vi "Teleop.vi"(10 "Match Info":T1={"Autonomous Elapsed Seconds"=0.0, "TeleOp Elapsed Seconds"=0.0, "Disabled Elapsed Seconds"=0.0, "Visited Autonomous"=FALSE, "Visited TeleOp"=FALSE, "Visited Disabled"=FALSE, "Autonomous Settings"={"Autonomous Style"=enum."Independent", "VI Refnum"=refnum}}, 11 "Call Context":T2) -> ()   [LabVIEW 2014]
doc: "This VI is called for each TeleOp packet received from the DS where the robot is not disabled. It is often used to read from the joysticks and update I/O or to update setpoints for timed control loops. It should complete and return within 20 milliseconds or it may miss DS packets."
uses:
  <vilib>/Rock Robotics/WPI/DriverStation/WPI_DriverStationDerivedRobotMode.ctl
  <vilib>/Rock Robotics/WPI/DriverStation/WPI_DriverStationMatch Info.ctl
  <vilib>/Rock Robotics/Network Tables/SD Read Boolean.vi
  <vilib>/Rock Robotics/Network Tables/SD Read Number.vi
  Global Var.vi
  <vilib>/Rock Robotics/WPI/Joystick/WPI_JoystickGetSetRefNum.vi
  <vilib>/addons/control/pid/pid.llb/PID (DBL).vi
  <vilib>/Rock Robotics/WPI/RobotDrive/WPI_RobotDriveGetSetRefNum.vi
  Global 1.vi
  <vilib>/Rock Robotics/Network Tables/SD Write Number.vi
  <vilib>/Rock Robotics/Network Tables/SD Write Boolean Array.vi
  <vilib>/Rock Robotics/Network Tables/SD Write Numeric Array.vi
  <vilib>/Rock Robotics/WPI/RobotDrive/WPI_RobotDriveMecanumDrive_Cartesian.vi
  <vilib>/addons/control/pid/NI_PID_pid.lvlib
panel:
  out "Sample Slider 0":dbl(slide) scale=0.0..5.0
  out "Sample Boolean 1":bool
  out "Sample Boolean 0":bool
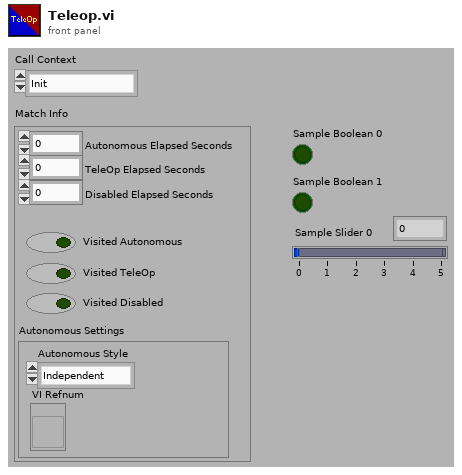
[diagram p1: front panel]
types:
  T1 = typedef "WPI_DriverStationMatch Info.ctl" = cluster{"Autonomous Elapsed Seconds":dbl, "TeleOp Elapsed Seconds":dbl, "Disabled Elapsed Seconds":dbl, "Visited Autonomous":bool, "Visited TeleOp":bool, "Visited Disabled":bool, "Autonomous Settings":cluster{"Autonomous Style":enum16{"Iterative", "Independent"}, "VI Refnum":refnum<vi>}}
  T2 = typedef "WPI_DriverStationDerivedRobotMode.ctl" = enum16{"Init", "Execute", "Stop"}
  T3 = typedef "WPI_JoystickDevRef.ctl" = cluster{"Device":T4}
  T4 = typedef "WPI_JoystickDeviceEnum.ctl" = enum16{"USB 0", "USB 1", "USB 2", "USB 3", "USB 4", "USB 5"}
  T5 = cluster{"Buttons[0]":bool, "Buttons[1]":bool, "Buttons[2]":bool, "Buttons[3]":bool, "Buttons[4]":bool, "Buttons[5]":bool, "Buttons[6]":bool, "Buttons[7]":bool, "Buttons[8]":bool, "Buttons[9]":bool, "Buttons[10]":bool, "Buttons[11]":bool}
  T6 = typedef "WPI_MotorControlDeviceRef.ctl" = cluster{"DeviceStatus":errorcluster, "Type":T7, "PWM":cluster{"Controller":T8, "PWM Channel":T9, "DeadBand":T10}, "CAN":cluster{"Device Number":u8, "Control Mode":T11, "Semaphore":T12, "Max Vout":dbl, "TalonSRX Control Mode":T13}, "Invert":bool, "TransformRef":T14, "InvTransformRef":T14}
  T7 = typedef "WPI_MotorControlType.ctl" = enum16{"PWM", "CAN", "CANTalonSRX"}
  T8 = typedef "FPGA_TypedefDigitalModule.ctl" = enum16{"Controller 1"}
  T9 = typedef "FPGA_DIOPWMChannel.ctl" = enum8{"PWM 0", "PWM 1", "PWM 2", "PWM 3", "PWM 4", "PWM 5", "PWM 6", "PWM 7", "PWM 8", "PWM 9", "PWM MXP 0", "PWM MXP 1", "PWM MXP 2", "PWM MXP 3", "PWM MXP 4", "PWM MXP 5", "PWM MXP 6", "PWM MXP 7", "PWM MXP 8", "PWM MXP 9", "Invalid"}
  T10 = typedef "WPI_PWMDeadband.ctl" = cluster{"Name":string, "maxPositivePwm":i32, "minPositivePwm":i32, "centerPwm":i32, "maxNegativePwm":i32, "minNegativePwm":i32, "angularRange":u16}
  T11 = typedef "WPI_CANJaguar_ControlMode.ctl" = enum8{"Percent VBus", "Current", "Speed", "Position", "Voltage"}
  T12 = typedef "Semaphore RefNum" = refnum<k1>
  T13 = typedef "WPI_CANTalonSRX_APIControlMode.ctl" = enum8{"Percent VBus", "Speed", "Position", "Slave", "Unchanged / Invalid"}
  T14 = typedef "WPI_PWMTransform_ConPane.ctl" = refnum<vi>
  T15 = typedef "WPI_RobotDriveDevRef.ctl" = cluster{"DevStatus":errorcluster, "Motors[]":T6[], "Square Inputs":bool, "Max Output":dbl}
  T16 = cluster{"proportional gain (Kc)":dbl, "integral time (Ti, min)":dbl, "derivative time (Td, min)":dbl}
  T17 = cluster{"Axes[0]":dbl, "Axes[1]":dbl, "Axes[2]":dbl, "Axes[3]":dbl, "Axes[4]":dbl, "Axes[5]":dbl, "Axes[6]":dbl, "Axes[7]":dbl, "Axes[8]":dbl, "Axes[9]":dbl, "Axes[10]":dbl, "Axes[11]":dbl}
  T18 = typedef "WPI_DigitalInputDevRef.ctl" = cluster{"DevStatus":errorcluster, "DIO Channel":T19, "Controller":T8}
  T19 = typedef "FPGA_DIOChannel.ctl" = enum8{"DIO 0", "DIO 1", "DIO 2", "DIO 3", "DIO 4", "DIO 5", "DIO 6", "DIO 7", "DIO 8", "DIO 9", "DIO MXP 0", "DIO MXP 1", "DIO MXP 2", "DIO MXP 3", "DIO MXP 4", "DIO MXP 5", "DIO MXP 6", "DIO MXP 7", "DIO MXP 8", "DIO MXP 9", "DIO MXP 10", "DIO MXP 11", "DIO MXP 12", "DIO MXP 13", "DIO MXP 14", "DIO MXP 15", "Invalid"}
  T20 = typedef "WPI_EncoderDevRef.ctl" = cluster{"DevStatus":errorcluster, "EncoderIndex":T21, "CounterIndex":T22, "DistancePerCount":dbl, "Decoding Type":T23}
  T21 = typedef "FPGA_EncoderIdx.ctl" = enum8{"Enc 0", "Enc 1", "Enc 2", "Enc 3", "Enc 4", "Enc 5", "Enc 6", "Enc 7", "Invalid"}
  T22 = typedef "FPGA_CounterCtrSystemIndex.ctl" = enum8{"Ctr 0", "Ctr 1", "Ctr 2", "Ctr 3", "Ctr 4", "Ctr 5", "Ctr 6", "Ctr 7", "Invalid"}
  T23 = typedef "WPI_EncoderType.ctl" = enum16{"1x", "2x", "4x"}
  T24 = cluster{"Buttons[0]":bool, "Buttons[1]":bool, "Buttons[2]":bool, "Buttons[3]":bool, "Buttons[4]":bool, "Buttons[5]":bool, "Buttons[6]":bool, "Buttons[7]":bool, "Buttons[8]":bool}
  T25 = typedef "WPI_GyroDevRef.ctl" = cluster{"DevStatus":errorcluster, "Analog Module":T26, "Analog Channel":T27, "Offset":dbl, "Gain (VoltsPerDegree/Second)":dbl}
  T26 = typedef "FPGA_TypedefAnalogModule.ctl" = enum16{"Controller 1"}
  T27 = typedef "FPGA_AIChannel.ctl" = enum8{"AI 0", "AI 1", "AI 2", "AI 3", "AI MXP 0", "AI MXP 1", "AI MXP 2", "AI MXP 3", "Invalid"}
  T28 = cluster{"Axes[0]":dbl, "Axes[1]":dbl, "Axes[2]":dbl, "Axes[3]":dbl, "Axes[4]":dbl, "Axes[5]":dbl, "Axes[6]":dbl, "Axes[7]":dbl, "Axes[8]":dbl}
  T29 = typedef "WPI_ServoDeviceRef.ctl" = cluster{"DeviceStatus":errorcluster, "Controller":T8, "PWM Channel":T9, "DeadBand":T10}
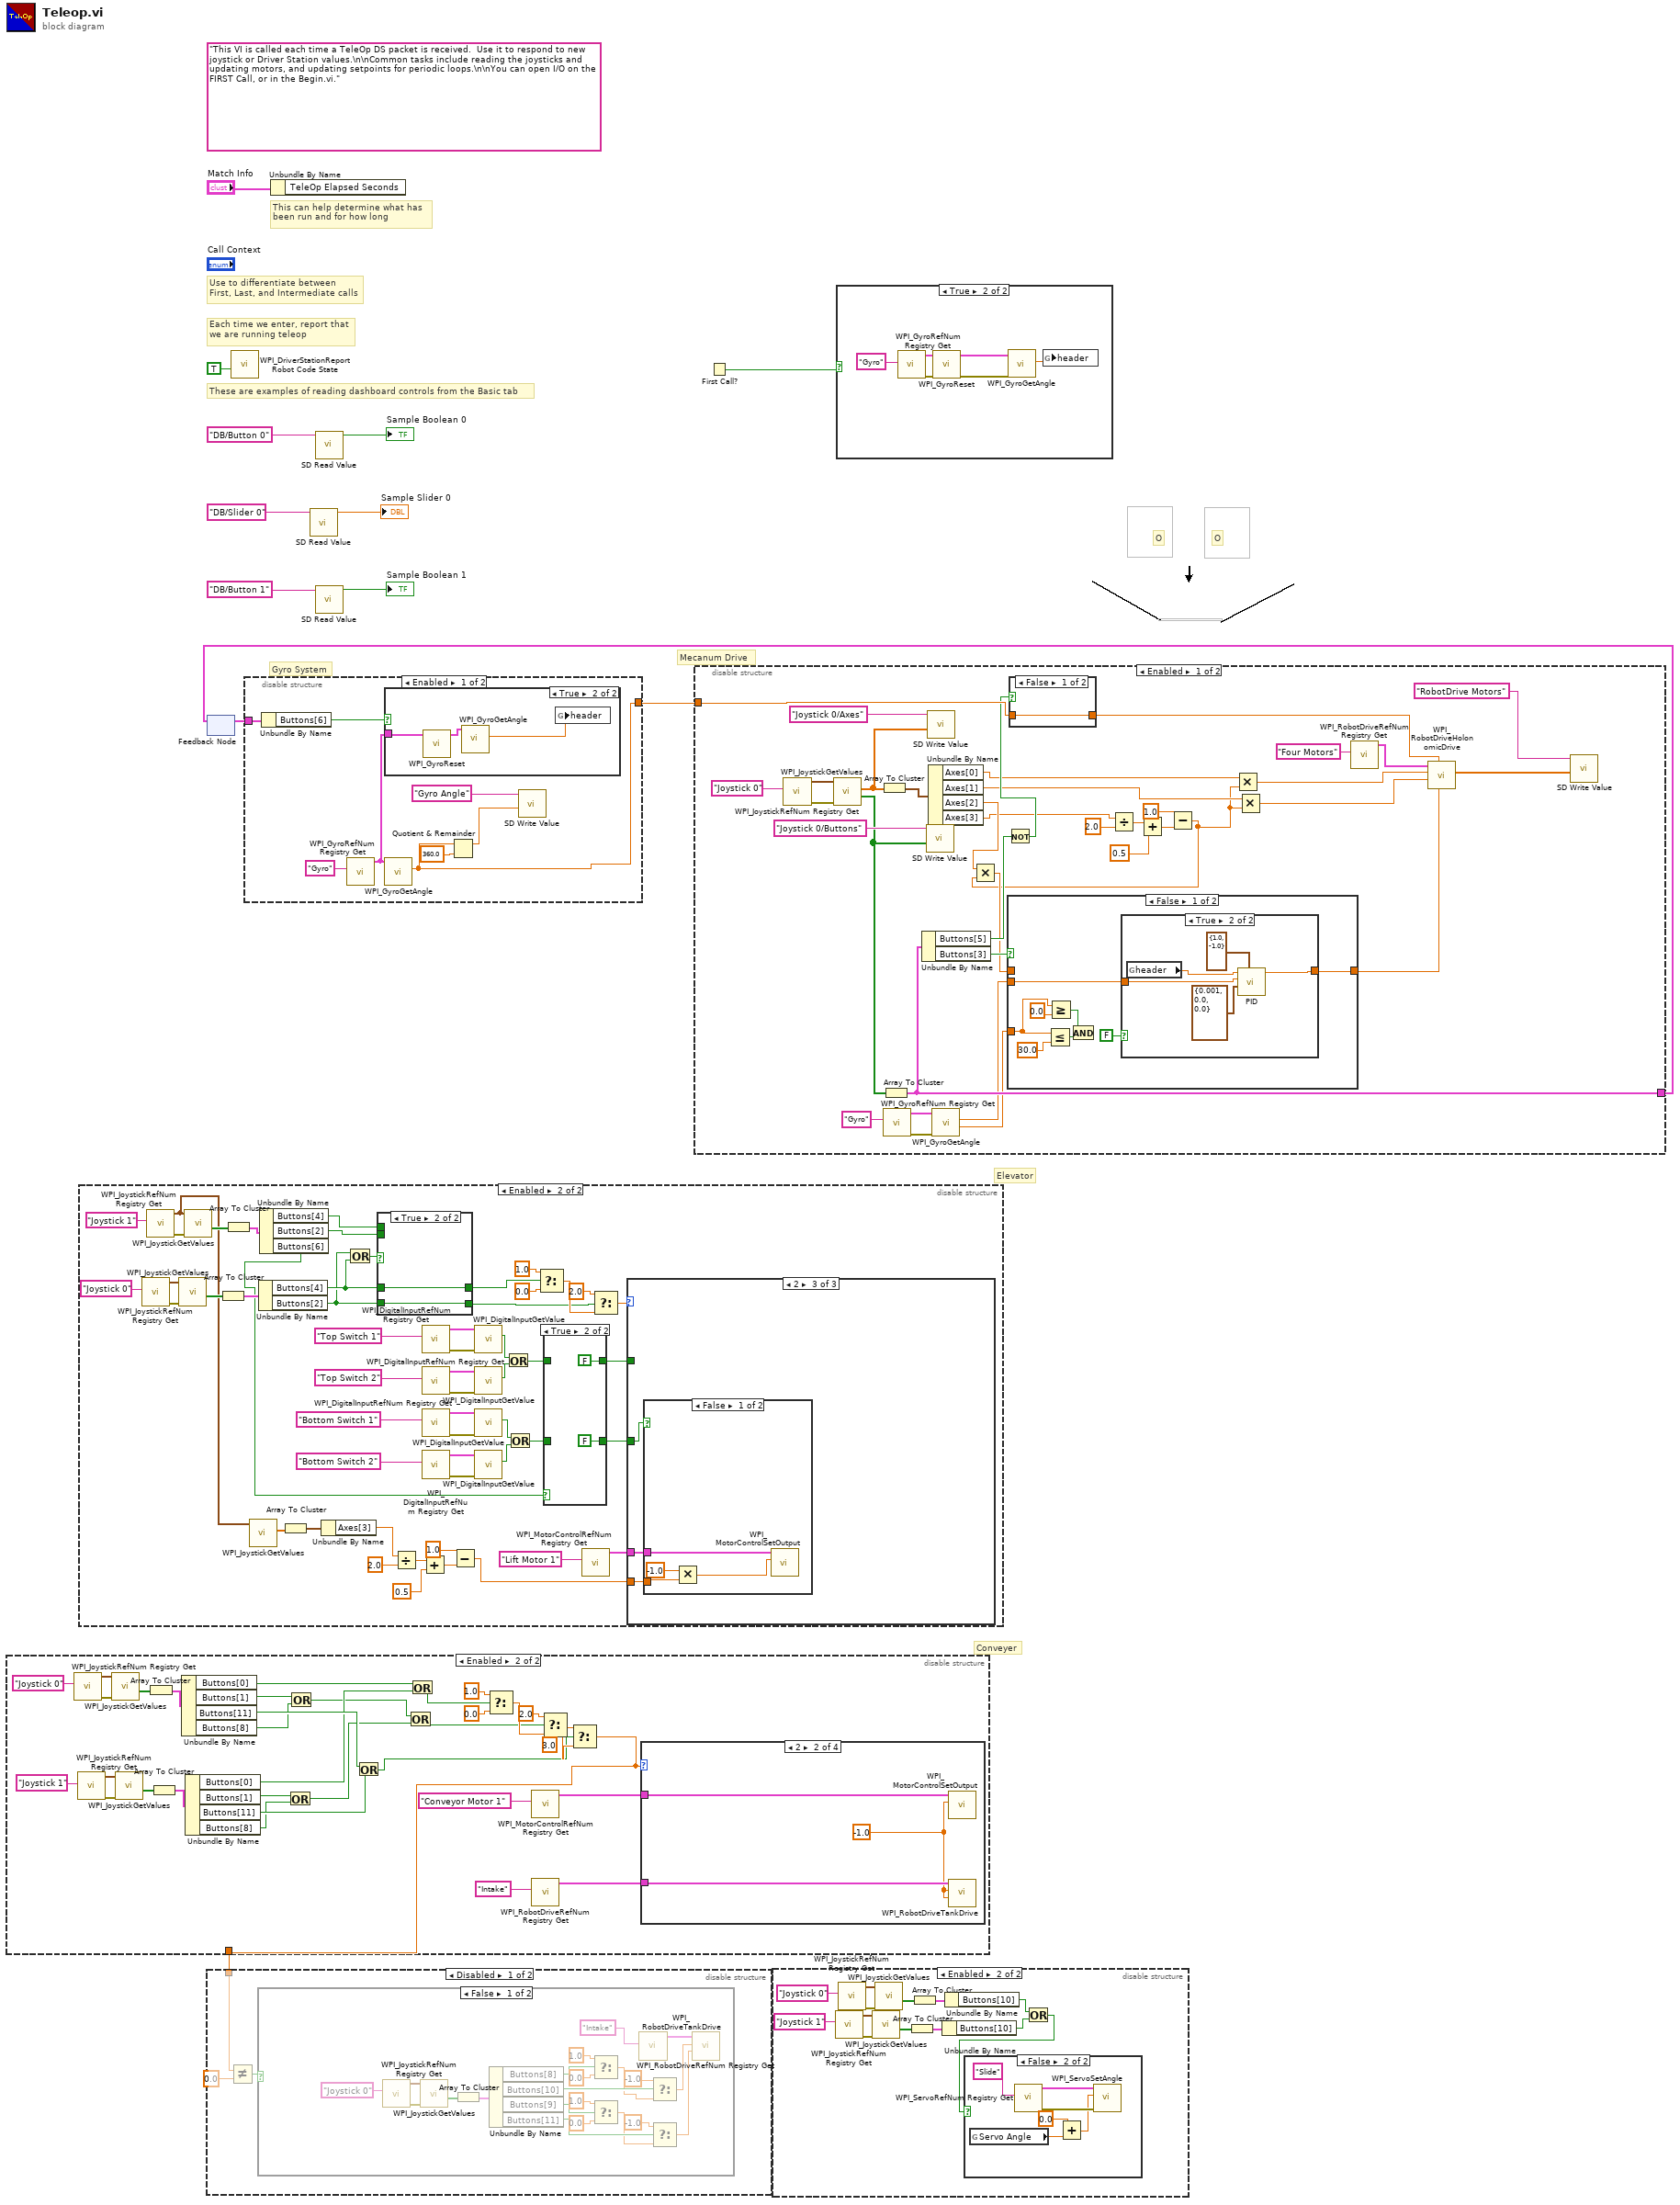
[diagram p0: block diagram]
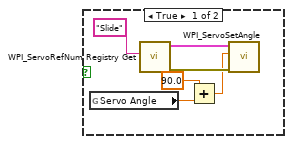
[diagram p3: hidden frame]
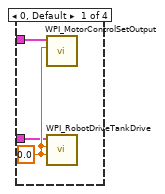
[diagram p8: hidden frame]
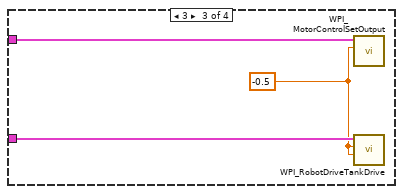
[diagram p9: hidden frame]
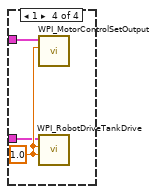
[diagram p10: hidden frame]
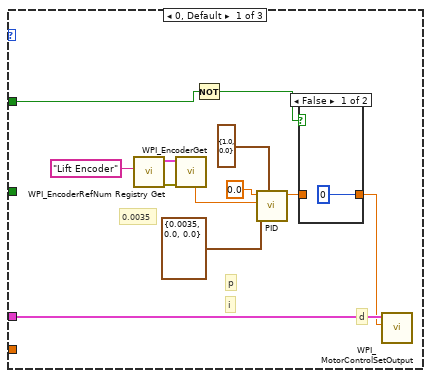
[diagram p14: hidden frame]
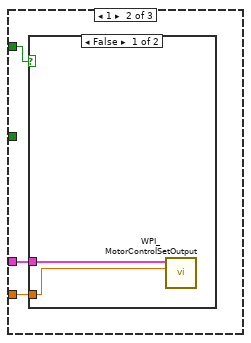
[diagram p16: hidden frame]
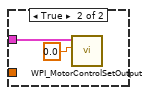
[diagram p17: hidden frame]
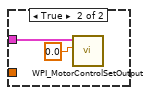
[diagram p18: hidden frame]
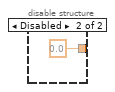
[diagram p20: hidden frame]
diagram:
  (unwired) "This VI is called each time a TeleOp DS packet is received.  Use it to respond to new joystick or Driver Station values.\n\nCommon tasks include reading the joysticks and updating motors, and updating setpoints for periodic loops.\n\nYou can open I/O on the FIRST Call, or in the Begin.vi."
  # "O"
  # "O"
  # "Conveyer"
  # "Gyro System"
  # "Mecanum Drive"
  # "Elevator"
  # "These are examples of reading dashboard controls from the Basic tab"
  # "Each time we enter, report that\nwe are running teleop"
  # "Use to differentiate between\nFirst, Last, and Intermediate calls"
  # "This can help determine what has\nbeen run and for how long"
  n1 = disable-structure shown="Enabled" {
    disable-tunnel: [_ w34] -> w1
    frame Disabled {
    }
    frame Enabled {
      n2 = call <vilib>:"WPI_JoystickRefNum Registry Get.vi"("refnum name"="Joystick 0") -> ("error out"=w43:errorcluster, "JoystickDevRef"=w44:T3)  [unwired: 9 in]
      n3 = call <vilib>:"WPI_JoystickRefNum Registry Get.vi"("refnum name"="Joystick 1") -> ("error out"=w29:errorcluster, "JoystickDevRef"=w30:T3)  [unwired: 9 in]
      n4 = call <vilib>:"WPI_JoystickGetValues.vi"("error in (no error)"=w43, "JoystickDevRef"=w44) -> ("Buttons"=w40:bool[])  [unwired: 5 in, 4 out]
      n5 = call <vilib>:"WPI_JoystickGetValues.vi"("error in (no error)"=w29, "JoystickDevRef"=w30) -> ("Buttons"=w28:bool[])  [unwired: 5 in, 4 out]
      n6 = Array To Cluster(array=w40) -> (cluster=w39:T5)
      n7 = Array To Cluster(array=w28) -> (cluster=w27:T5)
      n8 = Unbundle By Name(w39) -> ("Buttons[0]"=w20:bool, "Buttons[1]"=w17:bool, "Buttons[11]"=w24:bool, "Buttons[8]"=w18:bool)
      n9 = Unbundle By Name(w27) -> ("Buttons[0]"=w21:bool, "Buttons[1]"=w16:bool, "Buttons[11]"=w26:bool, "Buttons[8]"=w15:bool)
      n10 = Or(x=w16, y=w15) -> (x .or. y?=w14:bool)
      n11 = Or(x=w17, y=w18) -> (x .or. y?=w19:bool)
      n12 = Or(x=w24, y=w26) -> (x .or. y?=w25:bool)
      n13 = Or(x=w19, y=w14) -> (x .or. y?=w23:bool)
      n14 = Or(x=w20, y=w21) -> (x .or. y?=w22:bool)
      n15 = Select(t=1.0, s=w22, f=0.0) -> (s? t:f=w35:dbl)
      n16 = call <vilib>:"WPI_MotorControlRefNum Registry Get.vi"("refnum name"="Conveyor Motor 1") -> ("MotorControlDevRef"=w41:T6)  [unwired: 9 in, 1 out]
      n17 = call <vilib>:"WPI_RobotDriveRefNum Registry Get.vi"("refnum name"="Intake") -> ("RobotDriveDevRef"=w42:T15)  [unwired: 9 in, 1 out]
      n18 = Select(t=2.0, s=w23, f=w35) -> (s? t:f=w33:dbl)
      n19 = Select(t=3.0 ("f"), s=w25, f=w33) -> (s? t:f=w34:dbl)
      n20 = case shown="2" w34 {
        tunnel: w42 -> [w48 w52 w55 w57]
        tunnel: w41 -> [w50 w53 w56 w59]
        frame 0, Default {
          w49 = 0.0 ("Output")
          n21 = call <vilib>:"WPI_MotorControlSetOutput.vi"("Output"=w49, "MotorControlDevRef"=w50) -> ()  [unwired: 7 in, 3 out]
          n22 = call <vilib>:"WPI_RobotDriveTankDrive.vi"("Right axis value"=w49, "Left axis value"=w49, "RobotDriveDevRef"=w48) -> ()  [unwired: 6 in, 3 out]
        }
        frame 2 {
          w51 = -1.0
          n23 = call <vilib>:"WPI_MotorControlSetOutput.vi"("Output"=w51, "MotorControlDevRef"=w53) -> ()  [unwired: 7 in, 3 out]
          n24 = call <vilib>:"WPI_RobotDriveTankDrive.vi"("Right axis value"=w51, "Left axis value"=w51, "RobotDriveDevRef"=w52) -> ()  [unwired: 6 in, 3 out]
        }
        frame 3 {
          w54 = -0.5
          n25 = call <vilib>:"WPI_MotorControlSetOutput.vi"("Output"=w54, "MotorControlDevRef"=w56) -> ()  [unwired: 7 in, 3 out]
          n26 = call <vilib>:"WPI_RobotDriveTankDrive.vi"("Right axis value"=w54, "Left axis value"=w54, "RobotDriveDevRef"=w55) -> ()  [unwired: 6 in, 3 out]
        }
        frame 1 {
          w58 = 1.0 ("Output")
          n27 = call <vilib>:"WPI_MotorControlSetOutput.vi"("Output"=w58, "MotorControlDevRef"=w59) -> ()  [unwired: 7 in, 3 out]
          n28 = call <vilib>:"WPI_RobotDriveTankDrive.vi"("Right axis value"=w58, "Left axis value"=w58, "RobotDriveDevRef"=w57) -> ()  [unwired: 6 in, 3 out]
        }
      }
    }
  }
  n29 = disable-structure shown="Enabled" {
    frame Disabled {
    }
    frame Enabled {
      n30 = call <vilib>:"WPI_JoystickRefNum Registry Get.vi"("refnum name"="Joystick 0") -> ("error out"=w110:errorcluster, "JoystickDevRef"=w111:T3)  [unwired: 9 in]
      n31 = call <vilib>:"WPI_JoystickRefNum Registry Get.vi"("refnum name"="Joystick 1") -> ("error out"=w84:errorcluster, "JoystickDevRef"=w74:T3)  [unwired: 9 in]
      n32 = call <vilib>:"WPI_JoystickGetValues.vi"("error in (no error)"=w110, "JoystickDevRef"=w111) -> ("Buttons"=w102:bool[])  [unwired: 5 in, 4 out]
      n33 = call <vilib>:"WPI_JoystickGetValues.vi"("error in (no error)"=w84, "JoystickDevRef"=w74) -> ("Buttons"=w83:bool[])  [unwired: 5 in, 4 out]
      n34 = Array To Cluster(array=w102) -> (cluster=w101:T5)
      n35 = Array To Cluster(array=w83) -> (cluster=w82:T5)
      n36 = call <vilib>:"WPI_JoystickGetValues.vi"("JoystickDevRef"=w74) -> ("Axes"=w72:dbl[])  [unwired: 6 in, 4 out]
      n37 = Unbundle By Name(w101) -> ("Buttons[4]"=w76:bool, "Buttons[2]"=w75:bool)
      n38 = Unbundle By Name(w82) -> ("Buttons[4]"=w79:bool, "Buttons[2]"=w78:bool, "Buttons[6]"=w60:bool)
      n39 = Array To Cluster(array=w72) -> (cluster=w73:T17)
      n40 = Unbundle By Name(w73) -> ("Axes[3]"=w67:dbl)
      n41 = Or(x=w75, y=w76) -> (x .or. y?=w77:bool)
      n42 = case shown="True" w77 {
        tunnel: w76 -> [_ w121]
        tunnel: [w119 w121] -> w81
        tunnel: w75 -> [_ w120]
        tunnel: [w118 w120] -> w80
        tunnel: w79 -> [w119 _]
        tunnel: w78 -> [w118 _]
        frame False {
        }
        frame True {
        }
      }
      n43 = Divide(x=w67, y=2.0) -> (x/y=w70:dbl)
      n44 = Add(x=w70, y=0.5) -> (x+y=w69:dbl)
      n45 = call <vilib>:"WPI_DigitalInputRefNum Registry Get.vi"("refnum name"="Top Switch 1") -> ("error out"=w107:errorcluster, "DigitalInputDevRef"=w106:T18)  [unwired: 9 in]
      n46 = call <vilib>:"WPI_DigitalInputRefNum Registry Get.vi"("refnum name"="Top Switch 2") -> ("error out"=w91:errorcluster, "DigitalInputDevRef"=w90:T18)  [unwired: 9 in]
      n47 = call <vilib>:"WPI_DigitalInputRefNum Registry Get.vi"("refnum name"="Bottom Switch 1") -> ("error out"=w94:errorcluster, "DigitalInputDevRef"=w93:T18)  [unwired: 9 in]
      n48 = call <vilib>:"WPI_DigitalInputRefNum Registry Get.vi"("refnum name"="Bottom Switch 2") -> ("error out"=w104:errorcluster, "DigitalInputDevRef"=w103:T18)  [unwired: 9 in]
      n49 = Subtract(x=1.0, y=w69) -> (x-y=w65:dbl)
      n50 = call <vilib>:"WPI_DigitalInputGetValue.vi"("error in (no error)"=w107, "DigitalInputDevRef"=w106) -> ("Value"=w89:bool)  [unwired: 7 in, 2 out]
      n51 = call <vilib>:"WPI_DigitalInputGetValue.vi"("error in (no error)"=w91, "DigitalInputDevRef"=w90) -> ("Value"=w88:bool)  [unwired: 7 in, 2 out]
      n52 = call <vilib>:"WPI_DigitalInputGetValue.vi"("error in (no error)"=w94, "DigitalInputDevRef"=w93) -> ("Value"=w86:bool)  [unwired: 7 in, 2 out]
      n53 = call <vilib>:"WPI_DigitalInputGetValue.vi"("error in (no error)"=w104, "DigitalInputDevRef"=w103) -> ("Value"=w87:bool)  [unwired: 7 in, 2 out]
      n54 = Or(x=w89, y=w88) -> (x .or. y?=w61:bool)
      n55 = Or(x=w86, y=w87) -> (x .or. y?=w63:bool)
      n56 = Select(t=1.0, s=w81, f=0.0) -> (s? t:f=w96:dbl)
      n57 = case shown="True" w60 {
        tunnel: [w115 FALSE] -> w64
        tunnel: w63 -> [w115 _]
        tunnel: [w114 FALSE] -> w62
        tunnel: w61 -> [w114 _]
        frame False {
        }
        frame True {
        }
      }
      n58 = call <vilib>:"WPI_MotorControlRefNum Registry Get.vi"("refnum name"="Lift Motor 1") -> ("MotorControlDevRef"=w109:T6)  [unwired: 9 in, 1 out]
      n59 = Select(t=2.0, s=w80, f=w96) -> (s? t:f=w97:dbl)
      n60 = case shown="2" w97 {
        tunnel: w109 -> [w127 w138 w145]
        tunnel: w62 -> [w123 w137 _]
        tunnel: w64 -> [_ _ w144]
        tunnel: w65 -> [_ w136 w143]
        frame 0, Default {
          # "0.0035"
          # "d"
          # "i"
          # "p"
          n61 = call <vilib>:"WPI_EncoderRefNum Registry Get.vi"("refnum name"="Lift Encoder") -> ("error out"=w132:errorcluster, "EncoderDevRef"=w133:T20)  [unwired: 9 in]
          n62 = call <vilib>:"WPI_EncoderGet.vi"("error in (no error)"=w132, "EncoderDevRef"=w133) -> ("Rate"=w129:dbl)  [unwired: 4 in, 5 out]
          n63 = Not(x=w123) -> (.not. x?=w124:bool)
          n64 = call-poly <vilib>:"PID.vi"("output range"=cluster{"output high":dbl, "output low":dbl} {"output high"=1.0, "output low"=0.0}, "PID gains"=T16 {"proportional gain (Kc)"=0.0035, "integral time (Ti, min)"=0.0, "derivative time (Td, min)"=0.0}, "process variable"=w129, "setpoint"=0.0 ("Output")) -> ("output"=w125:dbl)  [unwired: 6 in, 1 out]
          n65 = case shown="False" w124 {
            tunnel: [0 w135] -> w126
            tunnel: w125 -> [_ w135]
            frame False {
            }
            frame True {
            }
          }
          n66 = call <vilib>:"WPI_MotorControlSetOutput.vi"("Output"=w126, "MotorControlDevRef"=w127) -> ()  [unwired: 7 in, 3 out]
        }
        frame 1 {
          n67 = case shown="False" w137 {
            tunnel: w138 -> [w140 w141]
            tunnel: w136 -> [w139 _]
            frame False {
              n68 = call <vilib>:"WPI_MotorControlSetOutput.vi"("Output"=w139, "MotorControlDevRef"=w140) -> ()  [unwired: 7 in, 3 out]
            }
            frame True {
              n69 = call <vilib>:"WPI_MotorControlSetOutput.vi"("Output"=0.0, "MotorControlDevRef"=w141) -> ()  [unwired: 7 in, 3 out]
            }
          }
        }
        frame 2 {
          n70 = case shown="False" w144 {
            tunnel: w145 -> [w149 w150]
            tunnel: w143 -> [w148 _]
            frame False {
              n71 = Multiply(x=-1.0, y=w148) -> (x*y=w147:dbl)
              n72 = call <vilib>:"WPI_MotorControlSetOutput.vi"("Output"=w147, "MotorControlDevRef"=w149) -> ()  [unwired: 7 in, 3 out]
            }
            frame True {
              n73 = call <vilib>:"WPI_MotorControlSetOutput.vi"("Output"=0.0, "MotorControlDevRef"=w150) -> ()  [unwired: 7 in, 3 out]
            }
          }
        }
      }
    }
  }
  n74 = feedback #1() -> (w5:T24)  [unwired: 1 in]
  n75 = disable-structure shown="Disabled" {
    disable-tunnel: w1 -> [w152 _]
    frame Disabled {
      n76 = Not Equal?(x=w152, y=0.0) -> (x != y?=w154:bool)
      n77 = case shown="False" w154 {
        frame False {
          n78 = call <vilib>:"WPI_JoystickRefNum Registry Get.vi"("refnum name"="Joystick 0") -> ("error out"=w172:errorcluster, "JoystickDevRef"=w171:T3)  [unwired: 9 in]
          n79 = call <vilib>:"WPI_JoystickGetValues.vi"("error in (no error)"=w172, "JoystickDevRef"=w171) -> ("Buttons"=w170:bool[])  [unwired: 5 in, 4 out]
          n80 = Array To Cluster(array=w170) -> (cluster=w169:T5)
          n81 = Unbundle By Name(w169) -> ("Buttons[8]"=w168:bool, "Buttons[10]"=w165:bool, "Buttons[9]"=w161:bool, "Buttons[11]"=w162:bool)
          n82 = Select(t=1.0, s=w168, f=0.0) -> (s? t:f=w157:dbl)
          n83 = Select(t=1.0, s=w161, f=0.0) -> (s? t:f=w158:dbl)
          n84 = call <vilib>:"WPI_RobotDriveRefNum Registry Get.vi"("refnum name"="Intake") -> ("RobotDriveDevRef"=w174:T15)  [unwired: 9 in, 1 out]
          n85 = Select(t=-1.0 ("f"), s=w165, f=w157) -> (s? t:f=w159:dbl)
          n86 = Select(t=-1.0 ("f"), s=w162, f=w158) -> (s? t:f=w160:dbl)
          n87 = call <vilib>:"WPI_RobotDriveTankDrive.vi"("Right axis value"=w160, "Left axis value"=w159, "RobotDriveDevRef"=w174) -> ()  [unwired: 6 in, 3 out]
        }
        frame True {
        }
      }
    }
    frame Enabled {
    }
  }
  n88 = call <vilib>:"WPI_DriverStationReport Robot Code State.vi"("TeleOp"=TRUE ("Autonomous")) -> ()  [unwired: 10 in, 1 out]
  n89 = disable-structure shown="Enabled" {
    disable-tunnel: w5 -> [w180 _]
    disable-tunnel: [w176 0.0] -> w4
    frame Enabled {
      n90 = Unbundle By Name(w180) -> ("Buttons[6]"=w179:bool)
      n91 = call <vilib>:"WPI_GyroRefNum Registry Get.vi"("refnum name"="Gyro") -> ("GyroDevRef"=w178:T25)  [unwired: 9 in, 1 out]
      n92 = case shown="True" w179 {
        tunnel: w178 -> [_ w186]
        frame False {
        }
        frame True {
          n93 = call <vilib>:"WPI_GyroReset.vi"("GyroDevRef"=w186) -> ("GyroDevRef"=w184:T25)  [unwired: 9 in, 1 out]
          n94 = call <vilib>:"WPI_GyroGetAngle.vi"("GyroDevRef"=w184) -> ("Angle"=w185:dbl)  [unwired: 7 in, 3 out]
          n95 = global write "Global Var.vi" "header"(w185) -> ()
        }
      }
      n96 = call <vilib>:"WPI_GyroGetAngle.vi"("GyroDevRef"=w178) -> ("Angle"=w176:dbl)  [unwired: 7 in, 3 out]
      n97 = Quotient & Remainder(x=w176, y=360.0) -> (x-y*floor(x/y)=w177:dbl)  [unwired: 1 out]
      n98 = call-poly <vilib>:"SD Write Value.vi"("Numeric"=w177, "Name"="Gyro Angle") -> ()  [unwired: 8 in, 2 out]
    }
    frame Disabled {
    }
  }
  n99 = Unbundle By Name("Match Info") -> ()  [unwired: 1 out]
  n100 = call-poly <vilib>:"SD Read Value.vi"("Name"="DB/Slider 0" ("refnum name")) -> ("Numeric"=→"Sample Slider 0":dbl)  [unwired: 8 in, 2 out]
  n101 = call-poly <vilib>:"SD Read Value.vi"("Name"="DB/Button 0" ("refnum name")) -> ("Boolean"=→"Sample Boolean 0":bool)  [unwired: 8 in, 2 out]
  n102 = call-poly <vilib>:"SD Read Value.vi"("Name"="DB/Button 1" ("refnum name")) -> ("Boolean"=→"Sample Boolean 1":bool)  [unwired: 8 in, 2 out]
  n103 = disable-structure shown="Enabled" {
    disable-tunnel: [w212 _] -> w3
    disable-tunnel: w4 -> [w205 _]
    frame Enabled {
      n104 = call <vilib>:"WPI_JoystickRefNum Registry Get.vi"("refnum name"="Joystick 0") -> ("error out"=w215:errorcluster, "JoystickDevRef"=w221:T3)  [unwired: 1 in, 8 out]
      n105 = call <vilib>:"WPI_JoystickGetValues.vi"("error in (no error)"=w215, "JoystickDevRef"=w221) -> ("Buttons"=w216:bool[], "Axes"=w214:dbl[])  [unwired: 5 in, 3 out]
      n106 = Array To Cluster(array=w214) -> (cluster=w213:T28)
      n107 = Array To Cluster(array=w216) -> (cluster=w212:T24)
      n108 = call <vilib>:"WPI_GyroRefNum Registry Get.vi"("refnum name"="Gyro") -> ("error out"=w208:errorcluster, "GyroDevRef"=w209:T25)  [unwired: 9 in]
      n109 = Unbundle By Name(w212) -> ("Buttons[5]"=w203:bool, "Buttons[3]"=w210:bool)
      n110 = call-poly <vilib>:"SD Write Value.vi"("Boolean Array"=w216, "Name"="Joystick 0/Buttons") -> ()  [unwired: 8 in, 2 out]
      n111 = call-poly <vilib>:"SD Write Value.vi"("Numeric Array"=w214, "Name"="Joystick 0/Axes") -> ()  [unwired: 8 in, 2 out]
      n112 = Unbundle By Name(w213) -> ("Axes[0]"=w196:dbl, "Axes[1]"=w198:dbl, "Axes[2]"=w194:dbl, "Axes[3]"=w192:dbl)
      n113 = call <vilib>:"WPI_GyroGetAngle.vi"("error in (no error)"=w208, "GyroDevRef"=w209) -> ("Angular Rate"=w206:dbl, "Angle"=w188:dbl)  [unwired: 6 in, 2 out]
      n114 = Not(x=w203) -> (.not. x?=w202:bool)
      n115 = case shown="False" w202 {
        tunnel: w205 -> [w225 _]
        tunnel: [w225 0.0 ("Angle")] -> w204
        frame False {
        }
        frame True {
        }
      }
      n116 = Divide(x=w192, y=2.0) -> (x/y=w200:dbl)
      n117 = Add(x=w200, y=0.5) -> (x+y=w190:dbl)
      n118 = Subtract(x=1.0, y=w190) -> (x-y=w191:dbl)
      n119 = Multiply(x=w194, y=w191) -> (x*y=w193:dbl)
      n120 = case shown="False" w210 {
        tunnel: [w234 w242] -> w211
        tunnel: w193 -> [_ w242]
        tunnel: w188 -> [w233 w241]
        tunnel: w206 -> [w230 _]
        frame False {
          n121 = Less Or Equal?(x=w230, y=30.0) -> (x <= y?=w228:bool)
          n122 = Greater Or Equal?(x=w230, y=0.0 ("x")) -> (x >= y?=w229:bool)
          n123 = And(x=w229, y=w228) -> ()  [unwired: 1 out]
          n124 = case shown="True" FALSE {
            tunnel: [0.0 ("output") w240] -> w234
            tunnel: w233 -> [_ w238]
            frame False {
            }
            frame True {
              n125 = global read "Global Var.vi" "header"() -> (w237:dbl)
              n126 = call-poly <vilib>:"PID.vi"("output range"=cluster{"output high":dbl, "output low":dbl} {"output high"=1.0, "output low"=-1.0}, "PID gains"=T16 {"proportional gain (Kc)"=0.001, "integral time (Ti, min)"=0.0, "derivative time (Td, min)"=0.0}, "process variable"=w238, "setpoint"=w237) -> ("output"=w240:dbl)  [unwired: 6 in, 1 out]
            }
          }
        }
        frame True {
          n127 = global write "Global Var.vi" "header"(w241) -> ()
        }
      }
      n128 = Multiply(x=w196, y=w191) -> (x*y=w195:dbl)
      n129 = Multiply(x=w198, y=w191) -> (x*y=w197:dbl)
      n130 = call <vilib>:"WPI_RobotDriveRefNum Registry Get.vi"("refnum name"="Four Motors") -> ("RobotDriveDevRef"=w223:T15)  [unwired: 1 in, 9 out]
      n131 = call-poly <vilib>:"WPI_RobotDriveHolonomicDrive.vi"("Rotation"=w211, "Gyro Angle"=w204, "Y"=w197, "X"=w195, "RobotDriveDevRef"=w223) -> ("Motor Values"=w217:dbl[])  [unwired: 4 in, 2 out]
      n132 = call-poly <vilib>:"SD Write Value.vi"("Numeric Array"=w217, "Name"="RobotDrive Motors") -> ()  [unwired: 8 in, 2 out]
    }
    frame Disabled {
    }
  }
  n133 = feedback-in #1(w3) -> ()
  n134 = First Call?() -> (First Call?: T/F=w2:bool)
  n135 = disable-structure shown="Enabled" {
    frame Disabled {
    }
    frame Enabled {
      n136 = call <vilib>:"WPI_JoystickRefNum Registry Get.vi"("refnum name"="Joystick 1") -> ("error out"=w253:errorcluster, "JoystickDevRef"=w254:T3)  [unwired: 9 in]
      n137 = call <vilib>:"WPI_JoystickRefNum Registry Get.vi"("refnum name"="Joystick 0") -> ("error out"=w248:errorcluster, "JoystickDevRef"=w249:T3)  [unwired: 9 in]
      n138 = call <vilib>:"WPI_JoystickGetValues.vi"("error in (no error)"=w253, "JoystickDevRef"=w254) -> ("Buttons"=w252:bool[])  [unwired: 5 in, 4 out]
      n139 = call <vilib>:"WPI_JoystickGetValues.vi"("error in (no error)"=w248, "JoystickDevRef"=w249) -> ("Buttons"=w247:bool[])  [unwired: 5 in, 4 out]
      n140 = Array To Cluster(array=w252) -> (cluster=w251:T5)
      n141 = Array To Cluster(array=w247) -> (cluster=w246:T5)
      n142 = Unbundle By Name(w251) -> ("Buttons[10]"=w245:bool)
      n143 = Unbundle By Name(w246) -> ("Buttons[10]"=w244:bool)
      n144 = Or(x=w244, y=w245) -> (x .or. y?=w243:bool)
      n145 = case shown="False" w243 {
        frame True {
          n146 = global read "Global 1.vi" "Servo Angle"() -> (w257:dbl)
          n147 = call <vilib>:"WPI_ServoRefNum Registry Get.vi"("refnum name"="Slide") -> ("error out"=w260:errorcluster, "ServoDeviceRef"=w259:T29)  [unwired: 9 in]
          n148 = Add(x=90.0, y=w257) -> (x+y=w256:dbl)
          n149 = call <vilib>:"WPI_ServoSetAngle.vi"("error in (no error)"=w260, "Angle"=w256, "ServoDeviceRef"=w259) -> ()  [unwired: 7 in, 2 out]
        }
        frame False {
          n150 = global read "Global 1.vi" "Servo Angle"() -> (w263:dbl)
          n151 = call <vilib>:"WPI_ServoRefNum Registry Get.vi"("refnum name"="Slide") -> ("error out"=w266:errorcluster, "ServoDeviceRef"=w265:T29)  [unwired: 9 in]
          n152 = Add(x=0.0, y=w263) -> (x+y=w262:dbl)
          n153 = call <vilib>:"WPI_ServoSetAngle.vi"("error in (no error)"=w266, "Angle"=w262, "ServoDeviceRef"=w265) -> ()  [unwired: 7 in, 2 out]
        }
      }
    }
  }
  n154 = case shown="True" w2 {
    frame False {
    }
    frame True {
      n155 = call <vilib>:"WPI_GyroRefNum Registry Get.vi"("refnum name"="Gyro") -> ("error out"=w271:errorcluster, "GyroDevRef"=w270:T25)  [unwired: 9 in]
      n156 = call <vilib>:"WPI_GyroReset.vi"("error in (no error)"=w271, "GyroDevRef"=w270) -> ("error out"=w268:errorcluster, "GyroDevRef"=w269:T25)  [unwired: 8 in]
      n157 = call <vilib>:"WPI_GyroGetAngle.vi"("error in (no error)"=w268, "GyroDevRef"=w269) -> ("Angle"=w272:dbl)  [unwired: 6 in, 3 out]
      n158 = global write "Global Var.vi" "header"(w272) -> ()
    }
  }
